vi "Read write template.vi"() -> ()   [LabVIEW 2012]
doc: "This VI shows how to use Network Streams to read data from one process and write to another."
uses:
  Datatype B.ctl
  Datatype A.ctl
  <vilib>/Platform/TimedLoop/XDataNode/timing_clust.ctl
  <vilib>/Platform/TimedLoop/XDataNode/nitl_modes.ctl
  <vilib>/Platform/TimedLoop/XDataNode/wakeup.ctl
  <vilib>/Instr/_visa.llb/VISA Configure Serial Port (Instr).vi
  <vilib>/Platform/TimedLoop/XDataNode/XDataNode.xnode
  <vilib>/Platform/TimedLoop/XDataNode/XDNodeRunTimeDep.lvlib
panel:
  out "read buffer":string
  in  "IMU Error":errorcluster
  in  "IMU VISA":refnum<visa-resource-name>
  in  "stop":bool
  out "Data A read":T1
  in  "Array of B Data":T2[](array[typedef])
  in  "Data A writer endpoint URL":string="//localhost/Data A Writer name"
  # "This example demonstrates how Network Streams could be used in a robotics application.  Examine the block diagrams of the example VIs to see the implementation.\n\nTo use this architecture, modify the data types according to what you need and update the URL's to point to the correct endpoint (changing localhost to the appropriate IP address, for example).  Then run the following VI's in any order:\nRead write template.vi\nWrite template.vi\nRead template.vi\n\nSee the readme.html for more help using this architecture with an RT Target."
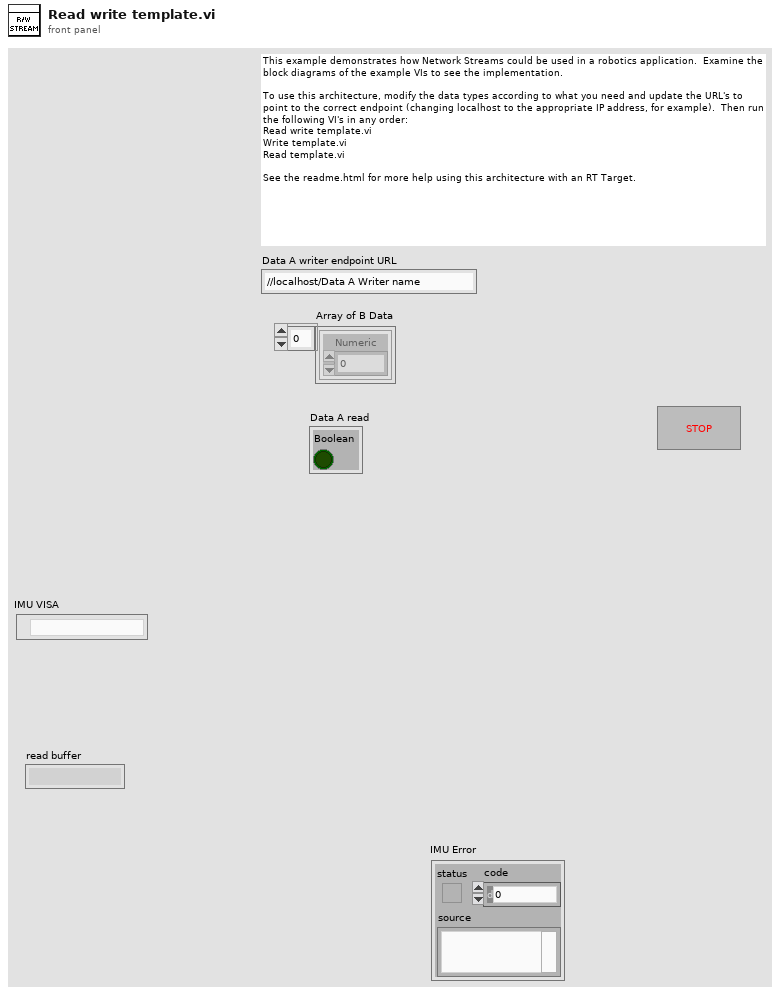
[diagram p1: front panel]
types:
  T1 = typedef "Datatype A.ctl" = cluster{"Boolean":bool}
  T2 = typedef "Datatype B.ctl" = cluster{"Numeric":dbl}
  T3 = typedef "XDNodeRunTimeDep.lvlib/timing_clust.ctl" = cluster{"Expected End [f-1]":u64, "Actual End [f-1]":u64, "Finished Late? [f-1]":bool, "Expected End [i-1]":u64, "Actual End [i-1]":u64, "Finished Late? [i-1]":bool, "Expected Start [i]":u64, "Actual Start [i]":u64, "Expected Start [f]":u64, "Actual Start [f]":u64, "Source Name":string, "Structure Name":string, "Period":i64, "Deadline":i64, "Offset":i64, "Start":i64, "Priority":i32, "Timeout":i32, "Mode":T4, "Wakeup Reason":T5, "Error":errorcluster, "Source Type":string, "Secondary Source Type":string, "Global End Time":u64, "Global Start Time":u64, "Frame Duration":u64, "Iteration Duration":u64, "Assigned CPU":i32, "I/O Scan Engine Mode":u32}
  T4 = typedef "XDNodeRunTimeDep.lvlib/nitl_modes.ctl" = enum32{"No Change", "Process missed periods, maintain original phase", "Discard missed periods, maintain original phase", "Process missed periods, ignore original phase", "Discard missed periods, ignore original phase"}
  T5 = typedef "XDNodeRunTimeDep.lvlib/wakeup.ctl" = enum32{"Normal", "Aborted", "Asynchronous wakeup", "Timing source error", "Timed loop error", "Timeout"}
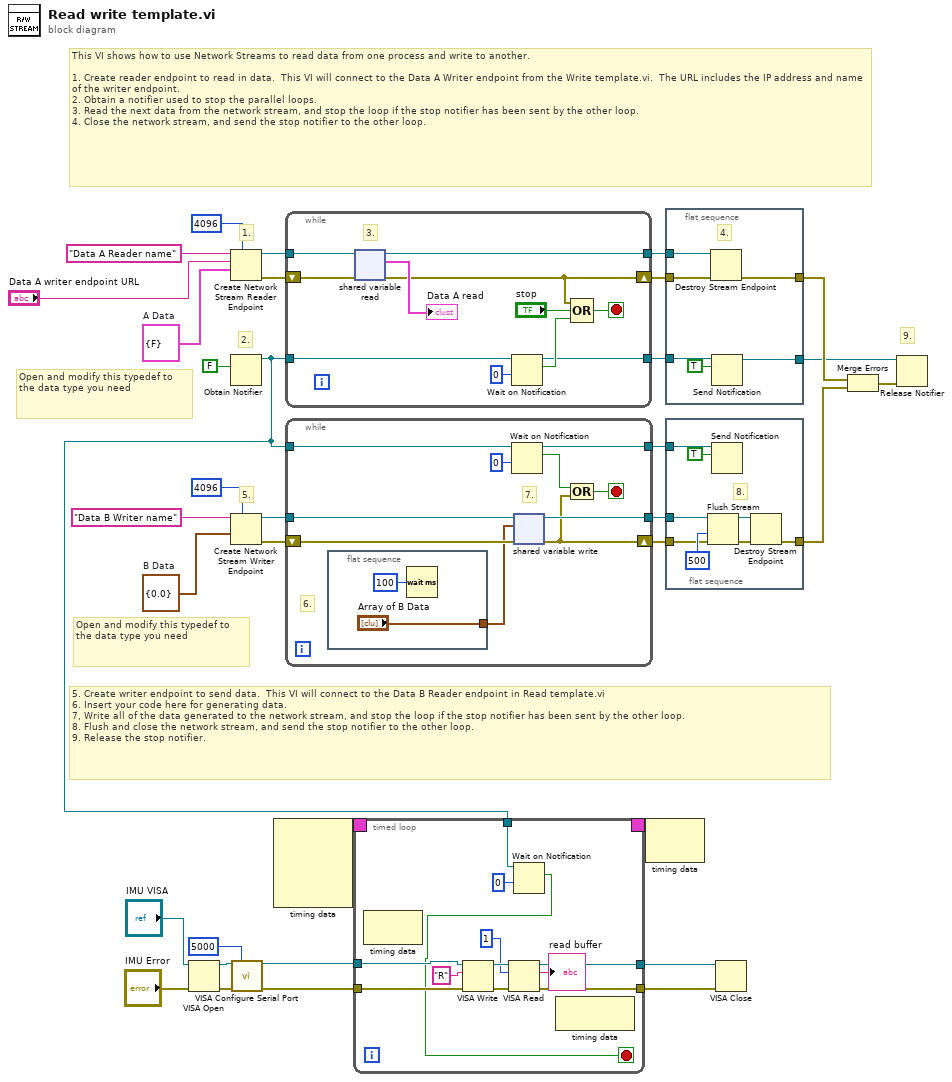
[diagram p0: block diagram]
diagram:
  w23 = T1 {"Boolean"=FALSE}  # A Data
  w24 = T2 {"Numeric"=0.0}  # B Data
  # "9."
  # "2."
  # "Open and modify this typedef to the data type you need"
  # "Open and modify this typedef to the data type you need"
  # "5."
  # "5. Create writer endpoint to send data.  This VI will connect to the Data B Reader endpoint in Read template.vi\n6. Insert your code here for generating data.\n7, Write all of the data generated to the network stream, and stop the loop if the stop notifier has been sent by the other loop.\n8. Flush and close the network stream, and send the stop notifier to the other loop.\n9. Release the stop notifier."
  # "1."
  # "This VI shows how to use Network Streams to read data from one process and write to another.  \n\n1. Create reader endpoint to read in data.  This VI will connect to the Data A Writer endpoint from the Write template.vi.  The URL includes the IP address and name of the writer endpoint.\n2. Obtain a notifier used to stop the parallel loops.\n3. Read the next data from the network stream, and stop the loop if the stop notifier has been sent by the other loop.\n4. Close the network stream, and send the stop notifier to the other loop."
  n1 = VISA Open(error in (no error)="IMU Error", VISA resource name="IMU VISA") -> (VISA resource name=w8:refnum<visa-resource-name>, error out=w9:errorcluster)  [unwired: 3 in]
  n2 = Create Network Stream Reader Endpoint(7:4096 ("reader buffer size"), 9:w23, 10:"Data A writer endpoint URL", 11:"Data A Reader name" ("reader name")) -> (0:w31:errorcluster, 3:w32:refnum<k21>)  [unwired: 3 in]
  n3 = Obtain Notifier(notification data type=FALSE) -> (notifier out=w1:refnum<notifier>)  [unwired: 3 in, 2 out]
  n4 = Create Network Stream Writer Endpoint(7:4096 ("writer buffer size"), 9:w24, 11:"Data B Writer name" ("writer name")) -> (0:w26:errorcluster, 3:w27:refnum<k21>)  [unwired: 4 in]
  n5 = call-poly "VISA Configure Serial Port"("VISA resource name"=w8, "timeout (10sec)"=u32 5000, "error in (no error)"=w9) -> ("VISA resource name out"=w5:refnum<visa-resource-name>, "error out"=w6:errorcluster)  [unwired: 11 in]
  n6 = node-c288() -> (w12:T3)  [unwired: 4 in]
  n7 = while {
    tunnel: w32 -> [w45]
    tunnel: [w43] -> w30
    tunnel: w1 -> [w39]
    tunnel: [w35] -> w20
    shift-right: [w36] -> w29
    shift-left: w31 -> [w44]
    stop <- w40 stop-if-true
    # "3."
    n8 = shared-variable-read(w45, w44) -> (w43:refnum<k21>, w36:errorcluster, →"Data A read":T1)  [unwired: 1 in, 1 out]
    n9 = Wait on Notification(notifier=w39, timeout in ms (-1)=0) -> (notifier out=w35:refnum<notifier>, notification=w37:bool)  [unwired: 2 in, 2 out]
    n10 = Compound Arithmetic op=OR(w36, "stop", w37) -> (w40:bool)
  }
  n11 = while {
    tunnel: w27 -> [w55]
    tunnel: [w54] -> w22
    tunnel: w1 -> [w50]
    tunnel: [w46] -> w19
    shift-right: [w49] -> w25
    shift-left: w26 -> [w53]
    stop <- w47 stop-if-true
    # "7."
    # "6."
    n12 = flat-sequence {
      tunnel: ["Array of B Data"] -> w52
      frame #0 {
        n13 = Wait (ms)(milliseconds to wait=u32 100) -> ()  [unwired: 1 out]
      }
    }
    n14 = Wait on Notification(notifier=w50, timeout in ms (-1)=0) -> (notifier out=w46:refnum<notifier>, notification=w48:bool)  [unwired: 2 in, 2 out]
    n15 = shared-variable-write(w55, w53, w52) -> (w54:refnum<k21>, w49:errorcluster)  [unwired: 1 in, 1 out]
    n16 = Compound Arithmetic op=OR(w48, w49) -> (w47:bool)
  }
  n17 = timed-loop {
    timing: w12 -> [_]
    timing-out: [_] -> w11
    tunnel: w6 -> [w69]
    tunnel: w5 -> [w68]
    tunnel: [w65] -> w4
    tunnel: [w64] -> w3
    tunnel: w1 -> [w59]
    stop <- w58 stop-if-true
    n18 = node-c288() -> ()  [unwired: 1 in, 1 out]
    n19 = VISA Write(VISA resource name=w68, write buffer="R", error in (no error)=w69) -> (VISA resource name out=w67:refnum<visa-resource-name>, error out=w66:errorcluster)  [unwired: 1 out]
    n20 = VISA Read(VISA resource name=w67, byte count=u32 1, error in (no error)=w66) -> (VISA resource name out=w64:refnum<visa-resource-name>, read buffer=→"read buffer":string, error out=w65:errorcluster)  [unwired: 1 out]
    n21 = Wait on Notification(notifier=w59, timeout in ms (-1)=0) -> (notification=w58:bool)  [unwired: 2 in, 3 out]
    n22 = node-c288() -> ()  [unwired: 1 in, 1 out]
  }
  n23 = node-c288(w11) -> ()  [unwired: 1 out]
  n24 = flat-sequence {
    tunnel: w30 -> [w77]
    tunnel: w29 -> [w76]
    tunnel: w20 -> [w75]
    tunnel: [w73] -> w18
    tunnel: [w72] -> w16
    frame #0 {
      # "4."
      n25 = Destroy Stream Endpoint(8:w76, 11:w77) -> (0:w73:errorcluster)
      n26 = Send Notification(notification=TRUE, notifier=w75) -> (notifier out=w72:refnum<notifier>)  [unwired: 1 in, 1 out]
    }
  }
  n27 = flat-sequence {
    tunnel: w25 -> [w82]
    tunnel: w22 -> [w81]
    tunnel: w19 -> [w79]
    tunnel: [w78] -> w17
    frame #0 {
      # "8."
      n28 = Flush Stream(8:w82, 9:500 ("timeout in ms (-1)"), 11:w81) -> (0:w85:errorcluster, 3:w84:refnum<k21>)  [unwired: 1 in, 1 out]
      n29 = Send Notification(notification=TRUE, notifier=w79) -> ()  [unwired: 1 in, 2 out]
      n30 = Destroy Stream Endpoint(8:w85, 11:w84) -> (0:w78:errorcluster)
    }
  }
  n31 = VISA Close(VISA resource name=w3, error in (no error)=w4) -> ()  [unwired: 1 out]
  n32 = Merge Errors(w18, w17) -> (w15:errorcluster)
  n33 = Release Notifier(notifier=w16, error in (no error)=w15) -> ()  [unwired: 1 in, 3 out]
